vi "Spartan HTTP File to Content-type.vi"(11 "file path":path=path "c:/web") -> (0 "using default type":bool, 1 "content-encoding":string, 2 "content-type":string, 3 "duplicate file path":path, 4 "extension":string, 6 "file name":string)   [LabVIEW 2011]
uses:
  Summitek EXT/OpenG EXT/file/file.llb/Strip Path Extension - Path__ogtk.vi
  ITK EXT/http/config.llb/HTTP SRM.vi
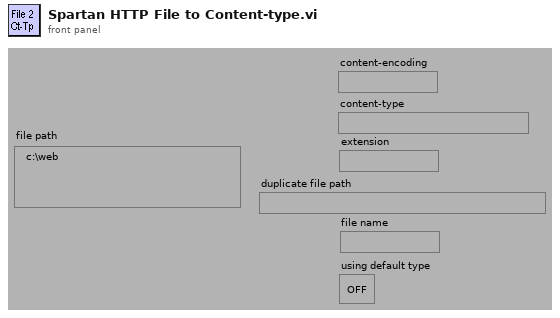
[diagram p1: front panel]
types:
  T1 = typedef "Keyed Array.ctl" = cluster{"keys":string[], "values":string[]}
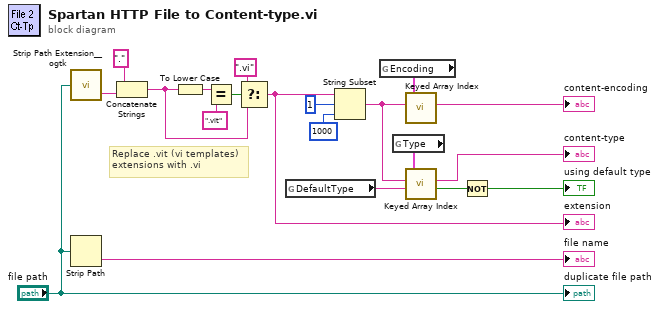
[diagram p0: block diagram]
diagram:
  # "Replace .vit (vi templates)\nextensions with .vi"
  n1 = call-poly "Strip Path Extension__ogtk.vi"("path"="file path") -> ("extension"=w2:string)  [unwired: 1 out]
  n2 = Strip Path(path="file path") -> (name=→"file name":string)  [unwired: 1 out]
  n3 = Concatenate Strings("." ("regular expression"), w2) -> (w1:string)
  n4 = To Lower Case(string=w1) -> (all lower case string=w8:string)
  n5 = Equal?(x=w8, y=".vit" ("regular expression")) -> (x = y?=w12:bool)
  n6 = Select(t=".vi" ("regular expression"), s=w12, f=w1) -> (s? t:f=w9:string)
  "extension" <- w9
  n7 = global read "HTTP SRM.vi" "DefaultType"() -> (w4:string)
  n8 = String Subset(string=w9, offset (0)=1, length (rest)=1000 ("length")) -> (substring=w15:string)
  n9 = global read "HTTP SRM.vi" "Encoding"() -> (w6:T1)
  n10 = global read "HTTP SRM.vi" "Type"() -> (w5:T1)
  n11 = call "Keyed Array Index.vi"("key"=w15, "array in"=w6) -> ("value"=→"content-encoding":string)  [unwired: 2 in, 3 out]
  n12 = call "Keyed Array Index.vi"("default value"=w4, "key"=w15, "array in"=w5) -> ("valid key"=w18:bool, "value"=→"content-type":string)  [unwired: 1 in, 2 out]
  n13 = Not(x=w18) -> (.not. x?=→"using default type":bool)
  "duplicate file path" <- "file path"
